vi "4155C PulsedStressV v2.0.vi"(0 "VISA resource name in":refnum<visa-resource-name>="GPIB0::14::INSTR", 1 "Gate":T1={"Gate Start"=10.0, "Gate Stop"=0.5, "Gate Step (linear only)"=1.0, "Gate Compliance"=0.001, "Gate PComp"=0.0, "Range mode"=0, "Range"=6} {"Range" max=11 scale=0.0..11.0; "Range mode" items=["Auto", "Limited", "Fixed"]; "Gate PComp" min=0.0 max=2.0 format="%^.2e"; "Gate Compliance" min=0.0 max=0.1 format="%^.2e"; "Gate Step (linear only)" min=-100.0 max=100.0 format="%^.4e"; "Gate Stop" min=-100.0 max=100.0 format="%^.4e"; "Gate Start" min=-100.0 max=100.0 format="%^.4e"}, 2 "Pulsed Stress V - Source/Common":u32(ring) items=["SMU1  ", "SMU2  ", "SMU3  ", "SMU4  ", "SMU5  ", "SMU6  "], 3 "Drain":T6={"Drain Start"=5.0, "Drain Stop"=2.0, "Drain Compliance"=0.001, "Drain Step"=1.0, "Drain PComp"=0.0, "Range mode"=0, "Range"=6} {"Range" max=11 scale=0.0..11.0; "Range mode" items=["Auto", "Limited", "Fixed"]; "Drain PComp" min=0.0 max=2.0 format="%^.2e"; "Drain Step" min=-100.0 max=100.0 format="%^.4e"; "Drain Compliance" min=0.0 max=0.1 format="%^.2e"; "Drain Stop" min=-100.0 max=100.0 format="%^.4e"; "Drain Start" min=-100.0 max=100.0 format="%^.4e"}, 4 "Timings":T5={"integration time"=0, "Short/Long integration time"=0.00064, "hold time (sec)"=0.0, "delay time (sec)"=0.0, "Step Time (0 disables)"=0.0, "sweep method"=0, "Pulse period"=0.1, "Base voltage"=0.0, "Pulse width"=0.05} {"Pulse width" min=0.0005 max=0.1 step=0.0001 format="%.4f"; "Base voltage" min=-100.0 max=100.0 format="%^.4e"; "Pulse period" min=0.005 max=1.0 step=0.0001 format="%.4f"; "sweep method" items=["Continuous", "Pulsed"]; "Step Time (0 disables)" min=0.0 format="%.2f"; "delay time (sec)" min=0.0 format="%.4f"; "hold time (sec)" min=0.0 format="%.4f"; "Short/Long integration time" min=0.0 format="%^.0e"; "integration time" scale=0.0..2.0}, 5 "error in (no error)":errorcluster, 6 "sweep mode":u16(ring) items=["Single", "Double"], 7 "Probe 4":cluster{"on/off":bool, "Voltage":dbl} {"Voltage" min=-100.0 max=100.0 format="%.2f"}, 8 "Pulsed Stress V - Drain":u32(ring)=1 items=["SMU1  ", "SMU2  ", "SMU3  ", "SMU4  ", "SMU5  ", "SMU6  "], 9 "Pulsed Stress V - Gate":u32(ring)=2 items=["SMU1  ", "SMU2  ", "SMU3  ", "SMU4  ", "SMU5  ", "SMU6  "], 10 "Panel Controls":T4={"Emergency Stop"=refnum, "TransGraph Max"=0.001, "Text/Graph (text=false)"=FALSE, "TransGraph Min"=1e-11} {"TransGraph Min" format="%.2e"; "TransGraph Max" format="%.2e"}, 11 "Standby":T2, 12 "Pulsed Stress V - Probe 4":u32(ring)=3 items=["SMU1  ", "SMU2  ", "SMU3  ", "SMU4  ", "SMU5  ", "SMU6  "], 15 "Pulsed Stress V - Vextra":u32(ring)=1 items=["VSU1  ", "VSU2  "]) -> (13 "Outparams":T3={"V2 Start"=0.0, "V2 Step"=0.0, "Number of points"=1} {"V2 Step" format="%.3f"; "V2 Start" format="%^.4e"}, 14 "VISA Resource Name out":refnum<visa-resource-name>, 17 "ID":dbl[](array[numeric]) format="%.2e", 18 "IG":dbl[](array[numeric]) format="%.2e", 19 "error out":errorcluster)   [LabVIEW 2016]
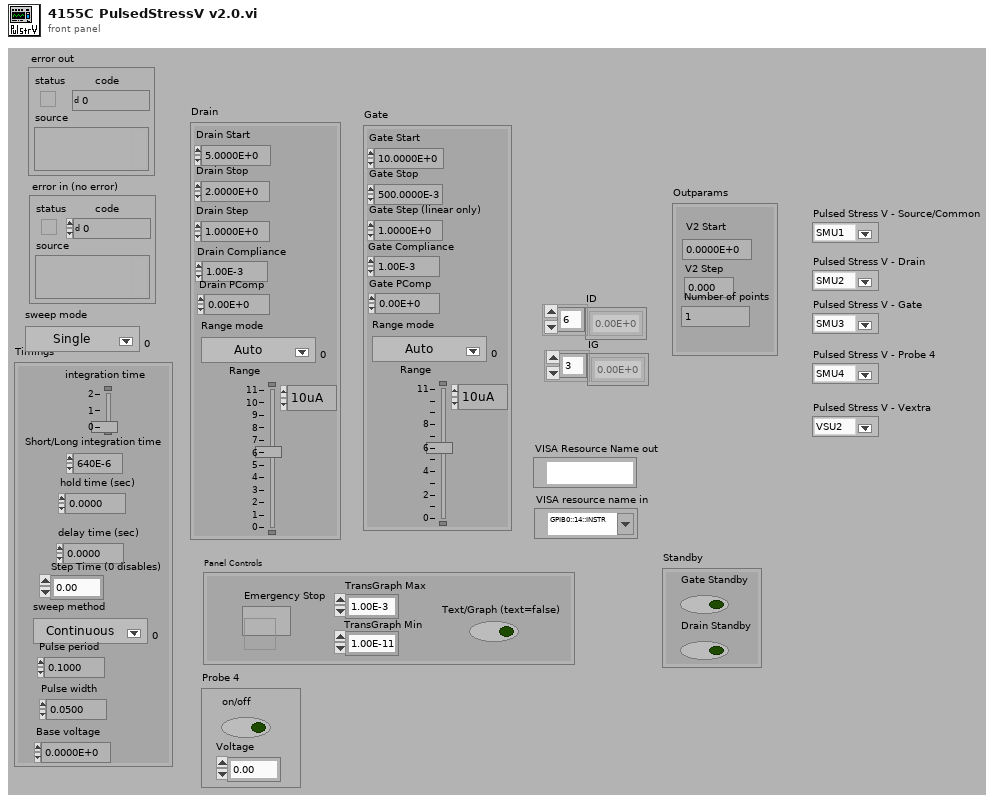
[diagram p1: front panel]
types:
  T1 = cluster{"Gate Start":dbl, "Gate Stop":dbl, "Gate Step (linear only)":dbl, "Gate Compliance":dbl, "Gate PComp":dbl, "Range mode":u16, "Range":u8}
  T2 = cluster{"Gate Standby":bool, "Drain Standby":bool}
  T3 = cluster{"V2 Start":dbl, "V2 Step":dbl, "Number of points":i32}
  T4 = cluster{"Emergency Stop":refnum<vi>, "TransGraph Max":dbl, "Text/Graph (text=false)":bool, "TransGraph Min":dbl}
  T5 = cluster{"integration time":u32, "Short/Long integration time":dbl, "hold time (sec)":dbl, "delay time (sec)":dbl, "Step Time (0 disables)":dbl, "sweep method":u16, "Pulse period":dbl, "Base voltage":dbl, "Pulse width":dbl}
  T6 = cluster{"Drain Start":dbl, "Drain Stop":dbl, "Drain Compliance":dbl, "Drain Step":dbl, "Drain PComp":dbl, "Range mode":u16, "Range":u8}
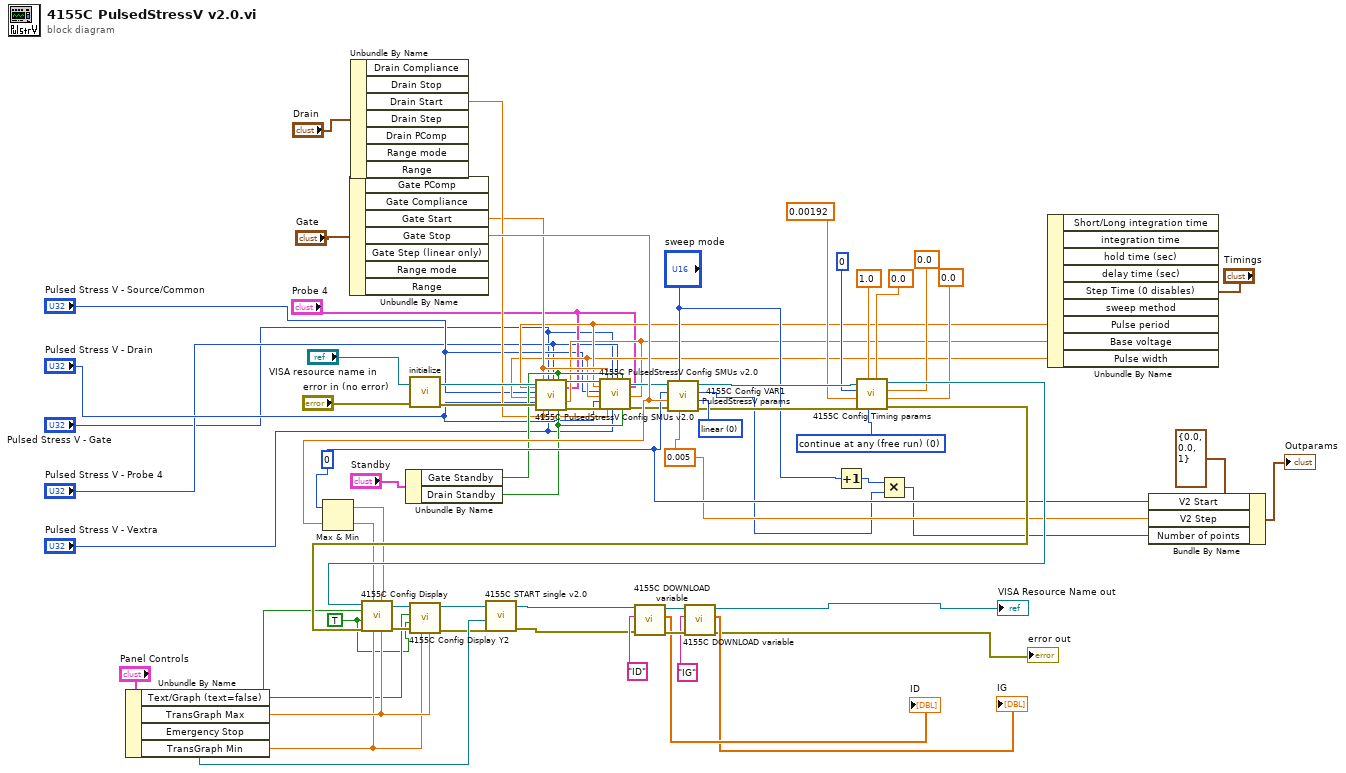
[diagram p0: block diagram]
diagram:
  w36 = 0.005 ("wait time parameter")
  w37 = 0
  w22 = TRUE ("Logarithmic")
  w63 = u8 0 items=["continue at any (free run)", "stop at any abnorm", "stop at compliance"] ("stop condition (free run:0)")
  w62 = u16 0 items=["linear", "log 10", "log 25", "log 50"] ("sweep spacing (linear: 0)")
  n1 = Unbundle By Name("Panel Controls") -> ("Text/Graph (text=false)"=w23:bool, "TransGraph Max"=w29:dbl, "Emergency Stop"=w56:refnum<vi>, "TransGraph Min"=w28:dbl)
  n2 = Unbundle By Name("Gate") -> ("Gate Start"=w10:dbl, "Gate Stop"=w43:dbl)  [unwired: 5 out]
  n3 = Max & Min(x=w37, y=w43) -> (max(x,y)=w30:dbl, min(x,y)=w31:dbl)
  n4 = Unbundle By Name("Drain") -> ("Drain Start"=w11:dbl)  [unwired: 6 out]
  n5 = Unbundle By Name("Standby") -> ("Gate Standby"=w13:bool, "Drain Standby"=w12:bool)
  n6 = call "initialize.vi"("error in (no error)"="error in (no error)", "VISA resource name in"="VISA resource name in") -> ("error out"=w19:errorcluster, "VISA Resource Name out"=w18:refnum<visa-resource-name>)
  n7 = Increment(x="sweep mode") -> (x+1=w33:u16)
  n8 = Unbundle By Name("Timings") -> ("Pulse period"=w9:dbl, "Base voltage"=w7:dbl, "Pulse width"=w8:dbl)  [unwired: 6 out]
  n9 = call "4155C PulsedStressV Config SMUs v2.0.vi"("VISA resource name in"=w18, "Pulse period"=w9, "Pulsed Stress V - Source/Common"="Pulsed Stress V - Source/Common", "Pulse width"=w8, "Pulsed Stress V - Drain"="Pulsed Stress V - Drain", "error in (no error)"=w19, "Gate ON voltage"=w10, "Drain Voltage"=w11, "Pulsed Stress V - Gate"="Pulsed Stress V - Gate", "Pulsed Stress V - Vextra"="Pulsed Stress V - Vextra", "Pulsed Stress V - Probe 4"="Pulsed Stress V - Probe 4", "Gate Standby"=w13, "Drain Standby"=w12, "Probe 4"="Probe 4", "Base voltage"=w7) -> ("VISA Resource Name out"=w14:refnum<visa-resource-name>, "error out"=w17:errorcluster)  [unwired: 3 in]
  n10 = call "4155C PulsedStressV Config SMUs v2.0.vi"("VISA resource name in"=w14, "Pulse period"=w9, "Pulsed Stress V - Source/Common"="Pulsed Stress V - Source/Common", "Pulse width"=w8, "Pulsed Stress V - Drain"="Pulsed Stress V - Drain", "error in (no error)"=w17, "Gate ON voltage"=w10, "Drain Voltage"=w11, "Pulsed Stress V - Gate"="Pulsed Stress V - Gate", "Pulsed Stress V - Vextra"="Pulsed Stress V - Vextra", "Pulsed Stress V - Probe 4"="Pulsed Stress V - Probe 4", "Gate Standby"=w13, "Drain Standby"=w12, "Probe 4"="Probe 4", "Base voltage"=w7) -> ("VISA Resource Name out"=w15:refnum<visa-resource-name>, "error out"=w16:errorcluster)  [unwired: 3 in]
  n11 = call "4155C Config VAR1 PulsedStressV params.vi"("sweep spacing (linear: 0)"=w62, "step (linear only)"=w36, "sweep mode"="sweep mode", "error in (no error)"=w16, "stop"=w43, "start"=w37, "VISA session"=w15) -> ("error out"=w44:errorcluster, "Number of points"=w34:i32, "dup VISA resource name"=w45:refnum<visa-resource-name>)  [unwired: 2 in]
  n12 = call "4155C Config Timing params.vi"("delay time (sec)"=0.0 ("wait time parameter"), "hold time (sec)"=0.0 ("wait time parameter"), "Step Time (0 disables)"=0.0 ("wait time parameter"), "stop condition (free run:0)"=w63, "wait time parameter"=1.0, "error in (no error)"=w44, "Short/Long integration time"=0.00192 ("wait time parameter"), "integration time"=0, "VISA session"=w45) -> ("error out"=w58:errorcluster, "dup VISA resource name"=w57:refnum<visa-resource-name>)  [unwired: 1 in]
  n13 = call "4155C Config Display.vi"("Ymax"=w29, "Var1 Stop"=w30, "Ymin"=w28, "Var1 Start"=w31, "error in (no error)"=w58, "Logarithmic"=w22, "SPA Display"=w23, "VISA session"=w57) -> ("error out"=w27:errorcluster, "dup VISA resource name"=w24:refnum<visa-resource-name>)  [unwired: 2 in]
  n14 = call "4155C Config Display Y2.vi"("Ymax"=w29, "Ymin"=w28, "error in (no error)"=w27, "Logarithmic"=w22, "SPA Display"=w23, "VISA session"=w24) -> ("error out"=w26:errorcluster, "dup VISA resource name"=w25:refnum<visa-resource-name>)  [unwired: 4 in]
  n15 = call "4155C START single v2.0.vi"("error in (no error)"=w26, "Emergency Stop"=w56, "VISA resource name in"=w25) -> ("error out"=w50:errorcluster, "VISA Resource Name out"=w51:refnum<visa-resource-name>)  [unwired: 3 in]
  n16 = call "4155C DOWNLOAD variable.vi"("error in (no error)"=w50, "Variable name"="ID", "VISA resource name in"=w51) -> ("error out"=w68:errorcluster, "Output data"=→"ID":dbl[], "VISA Resource Name out"=w67:refnum<visa-resource-name>)  [unwired: 2 in]
  n17 = call "4155C DOWNLOAD variable.vi"("error in (no error)"=w68, "Variable name"="IG", "VISA resource name in"=w67) -> ("error out"=→"error out":errorcluster, "Output data"=→"IG":dbl[], "VISA Resource Name out"=→"VISA Resource Name out":refnum<visa-resource-name>)  [unwired: 2 in]
  n18 = Multiply(x=w33, y=w34) -> (x*y=w32:i32)
  n19 = Bundle By Name(cluster=T3 {"V2 Start"=0.0, "V2 Step"=0.0, "Number of points"=1} ("Outparams"), "V2 Start"=w37, "V2 Step"=w36, "Number of points"=w32) -> (→"Outparams":T3)
